vi "Tester - read mic.vi"(8 "error in (no error)":errorcluster, 10 "Simulation Data":T1={"PowerOn"=TRUE, "Battery"=TRUE, "Antenna"=TRUE, "Microphone"=TRUE, "Speakers"=TRUE, "Buttons"=TRUE, "LCD"=enum."Passing Image"}, 11 "VISA resource name":refnum<visa-resource-name>) -> (0 "error out":errorcluster, 2 "Response Signal Out":waveform(dbl), 3 "VISA resource name out":refnum<visa-resource-name>)   [LabVIEW 2011]
uses:
  Simulation Data.ctl
  Audio Hardware Simulation Commands.ctl
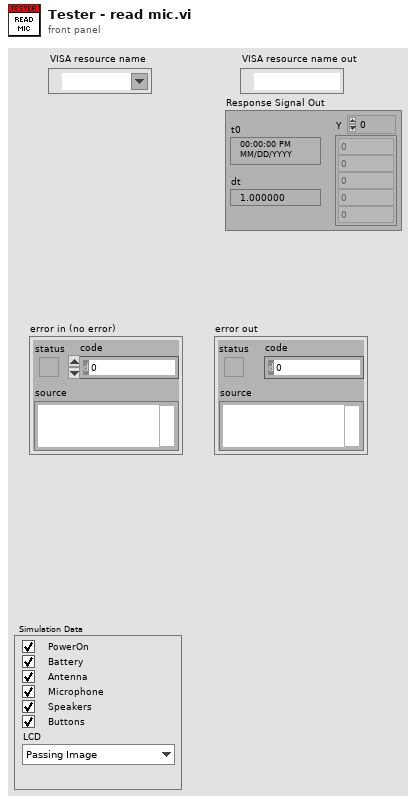
[diagram p1: front panel]
types:
  T1 = typedef "Simulation Data.ctl" = cluster{"PowerOn":bool, "Battery":bool, "Antenna":bool, "Microphone":bool, "Speakers":bool, "Buttons":bool, "LCD":enum16{"Passing Image", "Dead Pixels", "Incorrect Brightness"}}
  T2 = typedef "Audio Hardware Simulation Commands.ctl" = enum16{"Simulate Play Waveform", "Mic Test - Simulate Read Microphone", "Spkr Test - Simulate Read Microphone"}
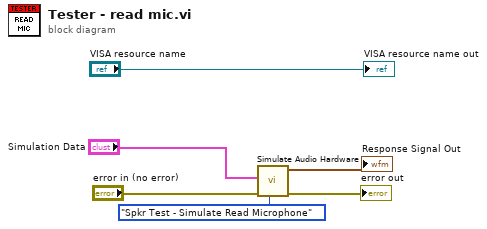
[diagram p0: block diagram]
diagram:
  n1 = call "Simulate Audio Hardware.vi"("Command to Simulate"=Audio_Hardware_Simulation_Commands."Spkr Test - Simulate Read Microphone", "error in (no error)"="error in (no error)", "Simulation Data"="Simulation Data") -> ("error out"=→"error out":errorcluster, "Response Signal Out"=→"Response Signal Out":waveform(dbl))  [unwired: 6 in]
  "VISA resource name out" <- "VISA resource name"
